vi "Init.vi"() -> (0 "Error Out":errorcluster, 3 "App Data Out":T4={"Console log"="", "GUI_Events"={"To_GUI-Producer"=refnum, "To_GUI-Error_message"=refnum, "To_GUI-msg_list"=refnum, "To_GUI-Session"=refnum, "To_GUI-Pre-Session"=refnum, "To_GUI-Consumer"=refnum}, "Function_Queue"={"Queue_MIDI_Handler"=refnum, "Queue_Session"=refnum, "Queue_Producer"=refnum, "Queue_Consumer"=refnum}, "Timout-Time[ms]"=0, "MIDI-Messages"=[], "Com Session State"=enum."Active Session", "Result Data"={"Diff"=[], "Tx Byte"=[], "Rx Byte"=[], "Send Log"=[], "Parsed Data"={"Tx MIDI Tag"=[], "Tx MIDI Parsed Data"=[], "Tx Error"=[], "Tx Running States"=[], "Rx MIDI Tag"=[], "Rx MIDI Parsed Data"=[], "Rx Error"=[], "Rx Running States"=[], "Diff"=[]}}, "Get #"=[], "CPU(ms)"=0})   [LabVIEW 2019]
doc: "Initialization of the software:\n- Setting initial values.\n- Loading initial files.\n\n1. Initialize all events\n2. Place events in the config cluster\n3. Initilizes all queues\n4. Place queue in config cluster\n5. Send Producer a message to initialize\n6. Set consumer type\n7. Set timeout Time \n\nEverything necessary before the GUI is running."
uses:
  Common/Controls/Application_Data.ctl
  Common/Controls/App_Events.ctl
  Common/Controls/App_Queues.ctl
  Common/Controls/Application_Message.ctl
  Common/Controls/Application_State.ctl
  MIDI/Controls/MIDI-Message_Array.ctl
  MIDI/Controls/MIDI-Message_Cluster.ctl
  MIDI/Controls/Meta_Commands.ctl
  Producer/Controls/Session_State.ctl
  Consumer/Controls/Consumer_Result.ctl
  Consumer/Controls/Parsed_Data.ctl
  <vilib>/Utility/error.llb/DialogType.ctl
panel:
  in  "Tab Control":T1(tab)
  out "Console Log":string
  in  "Function_Queue":T2
  in  "GUI_Events":T3
  in  "App Data":T4={"Console log"="", "GUI_Events"={"To_GUI-Producer"=refnum, "To_GUI-Error_message"=refnum, "To_GUI-msg_list"=refnum, "To_GUI-Session"=refnum, "To_GUI-Pre-Session"=refnum, "To_GUI-Consumer"=refnum}, "Function_Queue"={"Queue_MIDI_Handler"=refnum, "Queue_Session"=refnum, "Queue_Producer"=refnum, "Queue_Consumer"=refnum}, "Timout-Time[ms]"=0, "MIDI-Messages"=[], "Com Session State"=enum."Active Session", "Result Data"={"Diff"=[], "Tx Byte"=[], "Rx Byte"=[], "Send Log"=[], "Parsed Data"={"Tx MIDI Tag"=[], "Tx MIDI Parsed Data"=[], "Tx Error"=[], "Tx Running States"=[], "Rx MIDI Tag"=[], "Rx MIDI Parsed Data"=[], "Rx Error"=[], "Rx Running States"=[], "Diff"=[]}}, "Get #"=[], "CPU(ms)"=0}
  out "Error Message":string
  out "VI-filename":string
  out "VI Path":path
  in  "Execution:Show Front Panel On Call":bool
  in  "Tool Bar:Visible":bool
  out "Revision Number":u32
  out "Code Size":u32
  out "VI-Name":string
  # "Settings"
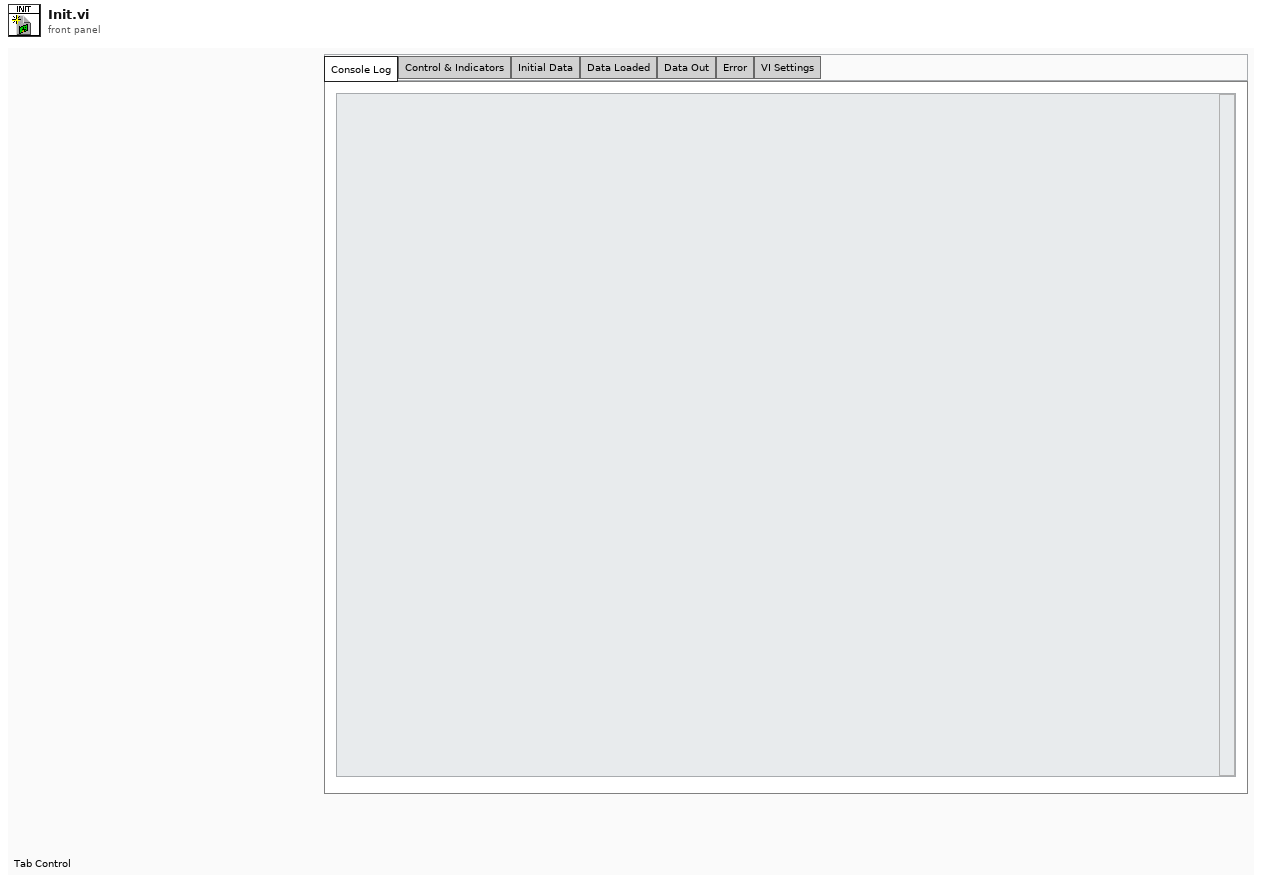
[diagram p1: front panel]
types:
  T1 = enum32{"Console Log", "Control & Indicators", "Initial Data", "Data Loaded", "Data Out", "Error", "VI Settings"}
  T2 = typedef "App_Queues.ctl" = cluster{"Queue_MIDI_Handler":refnum<queue>, "Queue_Session":refnum<queue>, "Queue_Producer":refnum<queue>, "Queue_Consumer":refnum<queue>}
  T3 = typedef "App_Events.ctl" = cluster{"To_GUI-Producer":refnum<user-event>, "To_GUI-Error_message":refnum<user-event>, "To_GUI-msg_list":refnum<user-event>, "To_GUI-Session":refnum<user-event>, "To_GUI-Pre-Session":refnum<user-event>, "To_GUI-Consumer":refnum<user-event>}
  T4 = typedef "Application_Data.ctl" = cluster{"Console log":string, "GUI_Events":T3, "Function_Queue":T2, "Timout-Time[ms]":i32, "MIDI-Messages":T5, "Com Session State":T8, "Result Data":T9, "Get #":bool[], "CPU(ms)":u32}
  T5 = typedef "MIDI-Message_Array.ctl" = T6[]
  T6 = typedef "MIDI-Message_Cluster.ctl" = cluster{"Message Name":string, "Meta value":i32, "Datastring":string, "Datatype":T7}
  T7 = typedef "Meta_Commands.ctl" = enum16{"No Data", "Pause", "Loop", "Wait for Rx", "Delay", "Break", "MIDI"}
  T8 = typedef "Session_State.ctl" = enum16{"Wait to begin", "Active Session", "Pause", "Wait for Response", "Stop", "Restart", "Inspect", "Exit"}
  T9 = typedef "Consumer_Result.ctl" = cluster{"Diff":bool[], "Tx Byte":string[], "Rx Byte":string[], "Send Log":string[], "Parsed Data":T10}
  T10 = typedef "Parsed_Data.ctl" = cluster{"Tx MIDI Tag":string[], "Tx MIDI Parsed Data":string[], "Tx Error":bool[], "Tx Running States":string[], "Rx MIDI Tag":string[], "Rx MIDI Parsed Data":string[], "Rx Error":bool[], "Rx Running States":string[], "Diff":bool[]}
  T11 = typedef "Application_Message.ctl" = cluster{"Application State":T12, "Payload":variant}
  T12 = typedef "Application_State.ctl" = enum16{"Idle", "Initiate", "MH Load Messages", "Prepare for Tx", "Settings", "Com Session", "Receive", "Data", "Uninitialize", "Quit Message", "Export Send"}
  T13 = typedef "DialogType.ctl" = u16
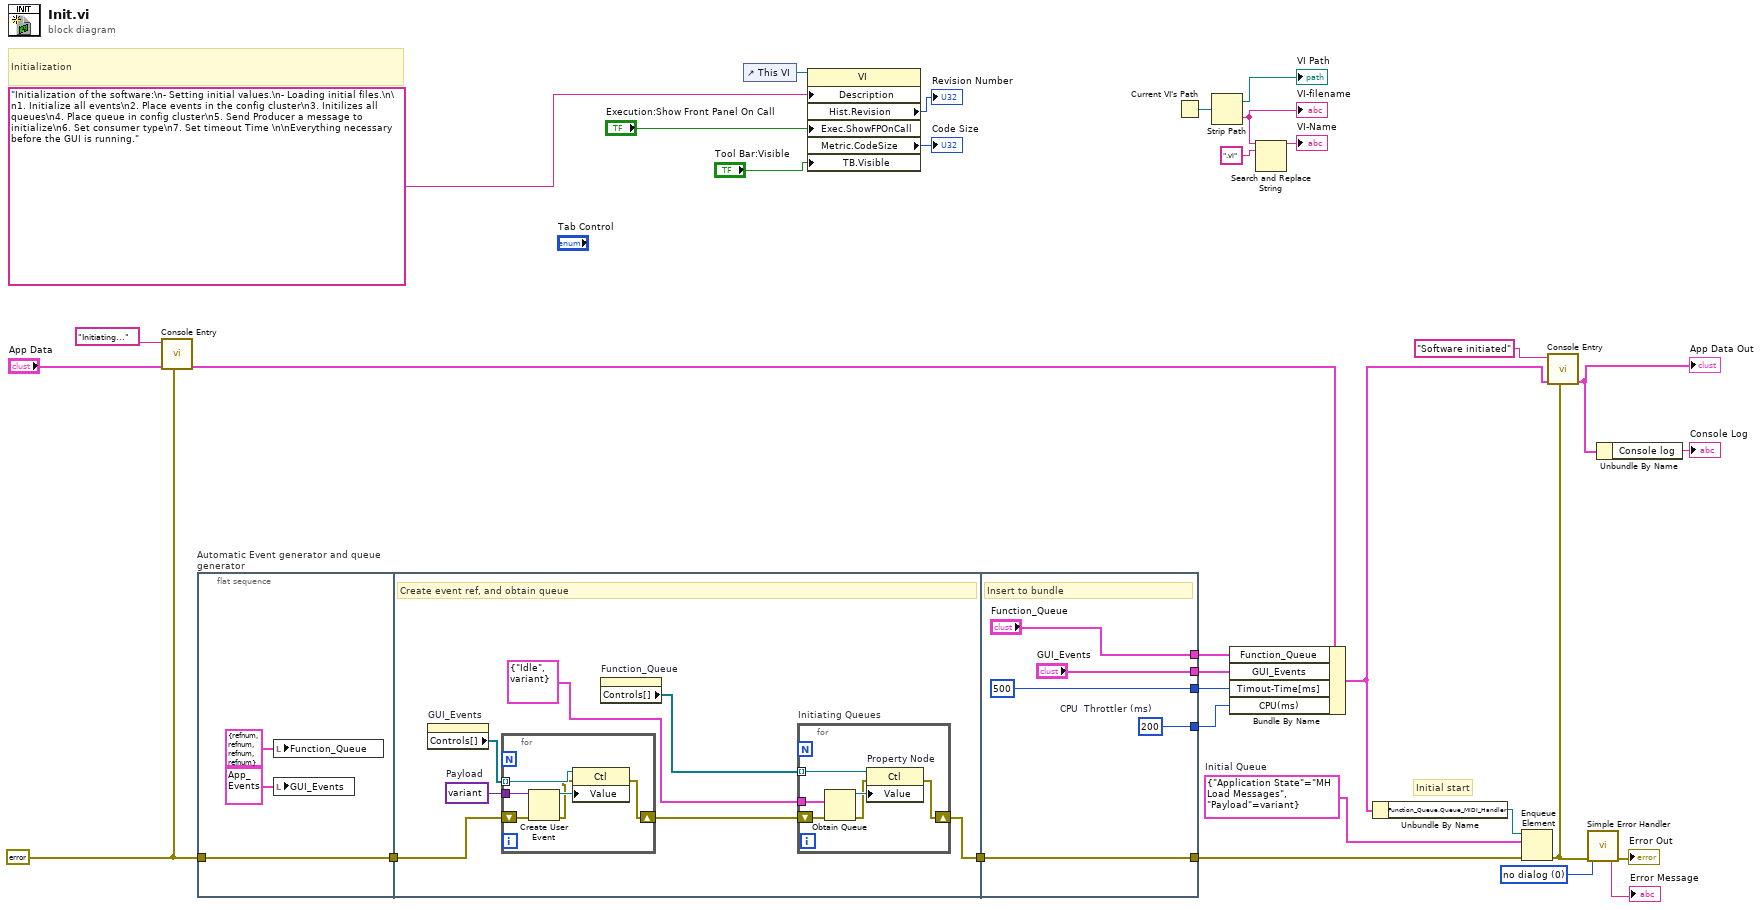
[diagram p0: block diagram]
diagram:
  w7 = T11 {"Application State"=enum."MH Load Messages", "Payload"=variant}  # Initial Queue
  w9 = T13 0 items=["no dialog", "OK message", "continue or stop message", "OK message + warnings", "continue/stop + warnings"] ("type of dialog (OK msg:1)")
  w2 = errorcluster {"status"=FALSE, "code"=0, "source"=""} ("Error Init")
  # "Initial start"
  # "Initialization"
  n1 = call "Console Entry.vi"("Error In"=w2, "Data In"="App Data", "Console Entry"="Initiating...") -> ("Data out"=w3:T4)  [unwired: 8 in]
  n2 = flat-sequence "Automatic Event generator and queue generator" {
    tunnel: [w35] -> w26
    tunnel: w2 -> [w35]
    tunnel: w26 -> [w42]
    tunnel: [w37] -> w25
    tunnel: [w59] -> w15
    tunnel: w25 -> [w59]
    tunnel: ["Function_Queue"] -> w24
    tunnel: ["GUI_Events"] -> w23
    tunnel: [500 ("Timout-Time[ms]")] -> w22
    tunnel: [w55] -> w5
    frame #0 {
      n3 = local write "Function_Queue"(T2 {"Queue_MIDI_Handler"=refnum, "Queue_Session"=refnum, "Queue_Producer"=refnum, "Queue_Consumer"=refnum} ("Function_Queue")) -> ()
      n4 = local write "GUI_Events"(T3 {"To_GUI-Producer"=refnum, "To_GUI-Error_message"=refnum, "To_GUI-msg_list"=refnum, "To_GUI-Session"=refnum, "To_GUI-Pre-Session"=refnum, "To_GUI-Consumer"=refnum} ("GUI_Events")) -> ()
    }
    frame #1 {
      w41 = variant  # Payload
      # "Create event ref, and obtain queue"
      n5 = property on="GUI_Events" class="Clust (strict)"() -> ("Controls[]"=w40:refnum<vi>[])  [unwired: 2 in, 2 out]
      n6 = for {
        shift-right: [w50] -> w38
        shift-left: w42 -> [w53]
        tunnel: w41 -> [w54]
        tunnel: w40 -> [w52] mode=indexing
        n7 = Create User Event(user event datatype=w54, error in=w53) -> (user event=w51:refnum<user-event>, error out=w49:errorcluster)
        n8 = property class="Ctl"(reference=w52, error in=w49, "Value"=w51) -> (error out=w50:errorcluster)  [unwired: 1 out]
      }
      n9 = property on="Function_Queue" class="Clust (strict)"() -> ("Controls[]"=w39:refnum<vi>[])  [unwired: 2 in, 2 out]
      n10 = for "Initiating Queues" {
        tunnel: w39 -> [w48] mode=indexing
        tunnel: T11 {"Application State"=enum."Idle", "Payload"=variant} ("Application Message") -> [w47]
        shift-right: [w43] -> w37
        shift-left: w38 -> [w46]
        n11 = Obtain Queue(element data type=w47, error in (no error)=w46) -> (queue out=w45:refnum<queue>, error out=w44:errorcluster)  [unwired: 3 in, 1 out]
        n12 = property on="Property Node" class="Ctl"(reference=w48, error in=w44, "Value"=w45) -> (error out=w43:errorcluster)  [unwired: 1 out]
      }
    }
    frame #2 {
      w55 = u32 200  # CPU  Throttler (ms)
      # "Insert to bundle"
    }
  }
  n13 = control-ref of="This VI"() -> (w14:refnum<vi>)
  n14 = property class="VI"(reference=w14, "Description"="Initialization of the software:\n- Setting initial values.\n- Loading initial files.\n\n1. Initialize all events\n2. Place events in the config cluster\n3. Initilizes all queues\n4. Place queue in config cluster\n5. Send Producer a message to initialize\n6. Set consumer type\n7. Set timeout Time \n\nEverything necessary before the GUI is running.", "Exec.ShowFPOnCall"="Execution:Show Front Panel On Call", "TB.Visible"="Tool Bar:Visible") -> ("Hist.Revision"=→"Revision Number":u32, "Metric.CodeSize"=→"Code Size":u32)  [unwired: 1 in, 2 out]
  n15 = Current VI's Path() -> (path=w32:path)
  n16 = Strip Path(path=w32) -> (stripped path=→"VI Path":path, name=w19:string)
  "VI-filename" <- w19
  n17 = Bundle By Name(cluster=w3, "Function_Queue"=w24, "GUI_Events"=w23, "Timout-Time[ms]"=w22, "CPU(ms)"=w5) -> (w12:T4)
  n18 = Search and Replace String(input string=w19, search string=".vi") -> (result string=→"VI-Name":string)  [unwired: 6 in, 3 out]
  n19 = Unbundle By Name(w12) -> ("Function_Queue.Queue_MIDI_Handler"=w21:refnum<queue>)
  n20 = Enqueue Element(queue=w21, element=w7, error in (no error)=w15) -> (error out=w10:errorcluster)  [unwired: 1 in, 2 out]
  n21 = call "Console Entry.vi"("Error In"=w10, "Data In"=w12, "Console Entry"="Software initiated" ("Console log")) -> ("Data out"=w13:T4)  [unwired: 8 in]
  "App Data Out" <- w13
  n22 = call <vilib>:"Simple Error Handler.vi"("type of dialog (OK msg:1)"=w9, "error in (no error)"=w10) -> ("error out"=→"Error Out":errorcluster, "message"=→"Error Message":string)  [unwired: 3 in, 3 out]
  n23 = Unbundle By Name(w13) -> ("Console log"=→"Console Log":string)
